vi "Actor Core.vi"(8 "error in":errorcluster, 11 "Nested in":refnum<class "MCLB_Template.lvclass">) -> (0 "error out":errorcluster, 3 "Actor out":refnum<class "Actor.lvclass">)   [LabVIEW 2021, in "MCLB_Template.lvclass"]
doc: "(<B>Filename</B>: Actor Framework.lvlib:Actor.lvclass:Actor Core.vi)\n\nReceives messages to the actor, reacts to them, and initiates any error handling that may shut the actor down.\n\nDescendant classes may override this VI to append parallel tasks for the actor to complete while it handles messages. Overrides use the Call Parent Method node."
uses:
  MCLB_Template.lvclass
  C:/Program Files (x86)/National Instruments/LabVIEW 2021/user.lib/John_Lib/AbstractActorTemplate/AbstractActorTemplate/UIActorTop.lvclass
  C:/Program Files (x86)/National Instruments/LabVIEW 2021/vi.lib/ActorFramework/Actor/Actor.lvclass
  <vilib>/ActorFramework/Actor/Actor.lvclass
  <userlib>/John_Lib/Control_Lib/MCLB_Lib/MCLB_Lib.lvclass
  <vilib>/Utility/miscctls.llb/LVRowAndColumnTypeDef.ctl
  MCLB_Template.lvclass/MCLB_Template.ctl
  <vilib>/ActorFramework/Actor/Actor.lvclass/Actor.ctl
  <vilib>/ActorFramework/Message Enqueuer/Message Enqueuer.lvclass/Message Enqueuer.ctl
  <vilib>/Utility/miscctls.llb/LVPoint32TypeDef.ctl
  <userlib>/John_Lib/Interfaces/MouseHandle Messages/Mouse Down Msg/Mouse Down Msg.lvclass/Mouse Down Msg.ctl
  <userlib>/John_Lib/Interfaces/MouseHandle Messages/Mouse RightDown Msg/Mouse RightDown Msg.lvclass/Mouse RightDown Msg.ctl
  <userlib>/John_Lib/Interfaces/Shortcut Menu Messages/Activation Msg/Activation Msg.lvclass/Activation Msg.ctl
  <userlib>/John_Lib/Interfaces/Shortcut Menu Messages/Menu Selection (User) Msg/Menu Selection (User) Msg.lvclass/Menu Selection (User) Msg.ctl
  <userlib>/John_Lib/Interfaces/MouseHandle Messages/Mouse Move Msg/Mouse Move Msg.lvclass/Mouse Move Msg.ctl
  <userlib>/John_Lib/Interfaces/MouseHandle Messages/Mouse UP Msg/Mouse UP Msg.lvclass/Mouse UP Msg.ctl
  <vilib>/ActorFramework/Message Enqueuer/Init from Existing Queue.vi
  <vilib>/ActorFramework/Message Enqueuer/Enqueue.vi
  <vilib>/ActorFramework/Stop Msg/Stop Msg.lvclass
  C:/Program Files (x86)/National Instruments/LabVIEW 2021/vi.lib/ActorFramework/Message/Message.lvclass
  <userlib>/John_Lib/Interfaces/MouseHandle Messages/Mouse Down Msg/Mouse Down Msg.lvclass
  <userlib>/John_Lib/Interfaces/MouseHandle Messages/Mouse RightDown Msg/Mouse RightDown Msg.lvclass
  <userlib>/John_Lib/Interfaces/Shortcut Menu Messages/Activation Msg/Activation Msg.lvclass
  <userlib>/John_Lib/Interfaces/Shortcut Menu Messages/Menu Selection (User) Msg/Menu Selection (User) Msg.lvclass
  <userlib>/John_Lib/Interfaces/MouseHandle Messages/Mouse Move Msg/Mouse Move Msg.lvclass
  <userlib>/John_Lib/Interfaces/MouseHandle Messages/Mouse UP Msg/Mouse UP Msg.lvclass
  <vilib>/ActorFramework/Message Priority Queue/Priority Enqueue.vi
  <vilib>/ActorFramework/Message Enqueuer/Message Enqueuer.lvclass
  <userlib>/John_Lib/AbstractActorTemplate/AbstractActorTemplate/UIActorTop.lvclass
panel:
  in  "MCLB":i32[](listbox)
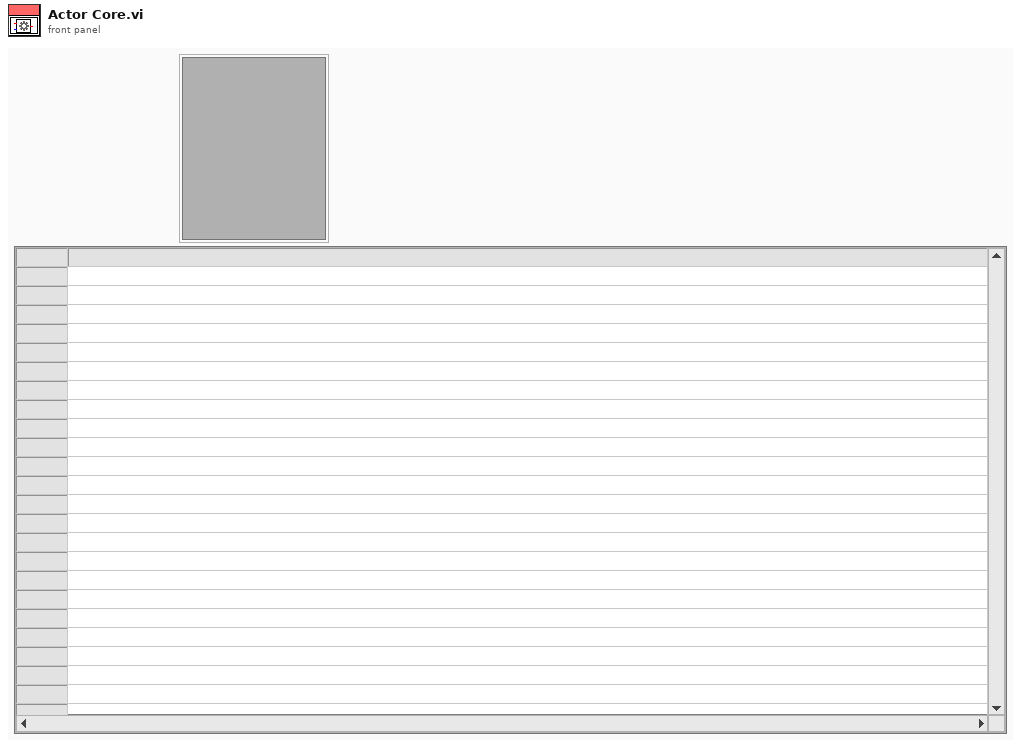
[diagram p1: front panel]
types:
  T1 = typedef "LVRowAndColumnTypeDef.ctl" = cluster{"Row":i32, "Column":i32}
  T2 = typedef "LVPoint32TypeDef.ctl" = cluster{"Horizontal":i32, "Vertical":i32}
  T3 = typedef "MouseButton.ctl" = enum16{"Idle", "Left", "Right", "Middle"}
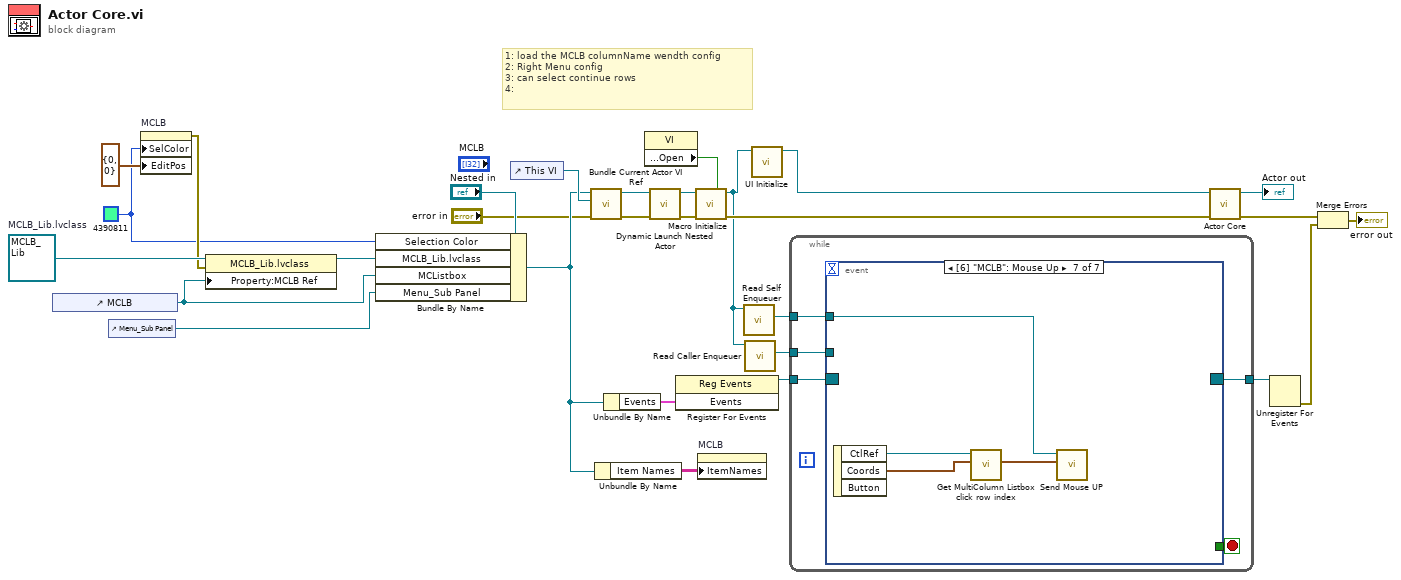
[diagram p0: block diagram]
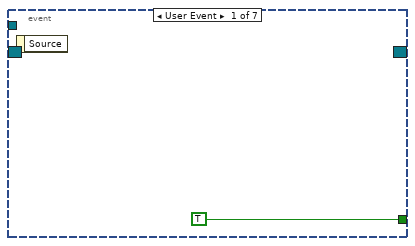
[diagram p2: hidden frame]
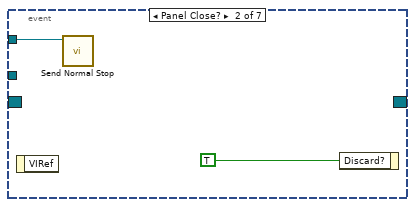
[diagram p3: hidden frame]
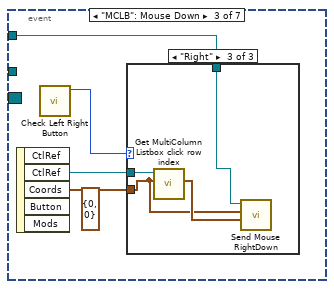
[diagram p4: hidden frame]
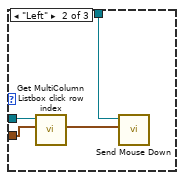
[diagram p6: hidden frame]
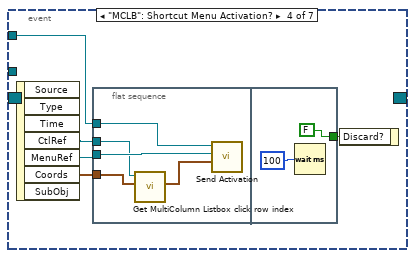
[diagram p7: hidden frame]
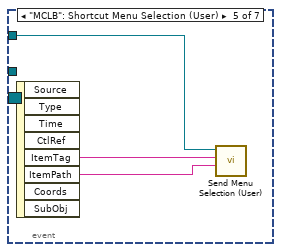
[diagram p8: hidden frame]
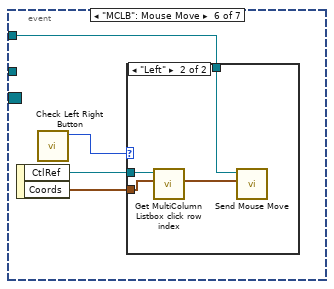
[diagram p9: hidden frame]
diagram:
  w12 = refnum<class "MCLB_Lib.lvclass"> refnum  # MCLB_Lib.lvclass
  w3 = u32 4390811 ("OK")
  # "1: load the MCLB columnName wendth config\n2: Right Menu config\n3: can select continue rows\n4:"
  n1 = control-ref of="MCLB"() -> (w10:refnum<vi>)
  n2 = control-ref of="Menu_Sub Panel"() -> (w9:refnum<vi>)
  n3 = property on="MCLB" class="MCListbox (strict)"("SelColor"=w3, "EditPos"=T1 {"Row"=0, "Column"=0} ("Edit Position")) -> (error out=w7:errorcluster)  [unwired: 2 in, 1 out]
  n4 = property class="MCLB_Lib.lvclass"(reference=w12, error in=w7, "Property:MCLB Ref"=w10) -> (reference out=w11:refnum<class "MCLB_Lib.lvclass">)  [unwired: 1 out]
  n5 = Bundle By Name(cluster="Nested in", "Selection Color"=w3, "MCLB_Lib.lvclass"=w11, "MCListbox"=w10, "Menu_Sub Panel"=w9) -> (w6:refnum<class "MCLB_Template.lvclass">)
  n6 = control-ref of="This VI"() -> (w13:refnum<vi>)
  n7 = call <userlib>:"Bundle Current Actor VI Ref.vi"("error in (no error)"="error in", "This VI"=w13, "UI ActorTop in"=w6) -> ("error out"=w14:errorcluster, "UI ActorTop out"=w15:refnum<class "MCLB_Template.lvclass">)  [unwired: 5 in, 2 out]
  n8 = Unbundle By Name(w6) -> ("Item Names"=w2:string[][])
  n9 = Unbundle By Name(w6) -> ("Events"=w27:cluster{"Stop":refnum<user-event>})
  n10 = property class="VI"() -> ("Front Panel.Open"=w22:bool)  [unwired: 2 in, 2 out]
  n11 = call-dynamic "Dynamic Launch Nested Actor.vi"("error in (no error)"=w14, "UI ActorTop in"=w15) -> ("error out"=w23:errorcluster, "UI ActorTop out"=w24:refnum<class "MCLB_Template.lvclass">)  [unwired: 8 in]
  n12 = register-events ("Main Register for Events")(w27) -> (reference out=w28:refnum<event-registration>)  [unwired: 2 in, 1 out]
  n13 = call-dynamic "Macro Initialize.vi"("Front Panel Window:Open"=w22, "error in (no error)"=w23, "UI ActorTop in"=w24) -> ("error out"=w18:errorcluster, "UI ActorTop out"=w5:refnum<class "MCLB_Template.lvclass">)  [unwired: 7 in]
  n14 = property on="MCLB" class="MCListbox (strict)"("ItemNames"=w2) -> ()  [unwired: 2 in, 2 out]
  n15 = call <vilib>:"Read Self Enqueuer.vi"("Actor"=w5) -> ("Self Enqueuer"=w25:refnum<class "Message Enqueuer.lvclass">)  [unwired: 10 in]
  n16 = call <vilib>:"Read Caller Enqueuer.vi"("Actor"=w5) -> ("Caller Enqueuer"=w17:refnum<class "Message Enqueuer.lvclass">)  [unwired: 10 in]
  n17 = call-dynamic "UI Initialize.vi"("UI ActorTop in"=w5) -> ("UI ActorTop out"=w4:refnum<class "MCLB_Template.lvclass">)  [unwired: 9 in, 1 out]
  n18 = while {
    tunnel: w28 -> [w34]
    tunnel: [w32] -> w26
    tunnel: w25 -> [w31]
    tunnel: w17 -> [w30]
    stop <- w33 stop-if-true
    n19 = event "UI Events" shown="[6] \"MCLB\": Mouse Up" {
      selector: w34 -> [_ _ _ _ _ _ _]
      dyn-events: [_ _ _ _ _ _ _] -> w32
      timeout: _ -> [_ _ _ _ _ _ _]
      tunnel: [TRUE _ _ _ _ _ _] -> w33
      tunnel: w31 -> [_ w36 w38 w54 w62 w65 w74]
      tunnel: w30 -> [_ _ _ _ _ _ _]
      event User Event {
        n20 = event-data() -> ()  [unwired: 1 in, 1 out]
      }
      event Panel Close? {
        n21 = event-data() -> ()  [unwired: 1 in, 1 out]
        n22 = call <vilib>:"Send Normal Stop.vi"("Message Enqueuer"=w36) -> ()  [unwired: 10 in, 1 out]
        n23 = event-data("Discard?"=TRUE) -> ()  [unwired: 1 in, 1 out]
      }
      event "MCLB": Mouse Down {
        (unwired) T2 {"Horizontal"=0, "Vertical"=0} ("Coords")
        n24 = event-data() -> ("CtlRef"=w41:refnum<vi>, "Coords"=w40:T2)  [unwired: 1 in, 3 out]
        n25 = call <userlib>:"Check Left Right Button.vi"() -> ("MouseButton"=w39:T3)  [unwired: 8 in, 3 out]
        n26 = case shown="\"Right\"" w39 {
          tunnel: w41 -> [_ w45 w49]
          tunnel: w40 -> [_ w44 w46]
          tunnel: w38 -> [_ w42 w48]
          frame "Idle", Default {
          }
          frame "Left" {
            n27 = call <userlib>:"Get MultiColumn Listbox click row index.vi"("Coords"=w44, "CtlRef"=w45) -> ("Cell Position"=w43:T1)  [unwired: 5 in, 4 out]
            n28 = call <userlib>:"Send Mouse Down.vi"("Cell Position"=w43, "Message Enqueuer"=w42) -> ()  [unwired: 8 in, 2 out]
          }
          frame "Right" {
            n29 = call <userlib>:"Get MultiColumn Listbox click row index.vi"("Coords"=w46, "CtlRef"=w49) -> ("Cell Position"=w47:T1)  [unwired: 5 in, 4 out]
            n30 = call <userlib>:"Send Mouse RightDown.vi"("Cell Position"=w47, "Coords"=w46, "Message Enqueuer"=w48) -> ()  [unwired: 7 in, 2 out]
          }
        }
      }
      event "MCLB": Shortcut Menu Activation? {
        n31 = event-data() -> ("CtlRef"=w50:refnum<vi>, "MenuRef"=w53:refnum<k9>, "Coords"=w51:T2)  [unwired: 1 in, 4 out]
        n32 = flat-sequence {
          tunnel: w54 -> [w59]
          tunnel: w53 -> [w56]
          tunnel: w51 -> [w57]
          tunnel: w50 -> [w55]
          tunnel: [FALSE ("Discard?")] -> w52
          frame #0 {
            n33 = call <userlib>:"Get MultiColumn Listbox click row index.vi"("Coords"=w57, "CtlRef"=w55) -> ("Cell Position"=w58:T1)  [unwired: 5 in, 4 out]
            n34 = call <userlib>:"Send Activation.vi"("Cell Position"=w58, "MenuRef"=w56, "Message Enqueuer"=w59) -> ()  [unwired: 7 in, 2 out]
          }
          frame #1 {
            n35 = Wait (ms)(milliseconds to wait=u32 100) -> ()  [unwired: 1 out]
          }
        }
        n36 = event-data("Discard?"=w52) -> ()  [unwired: 1 in, 1 out]
      }
      event "MCLB": Shortcut Menu Selection (User) {
        n37 = event-data() -> ("ItemTag"=w63:string, "ItemPath"=w64:string)  [unwired: 1 in, 6 out]
        n38 = call <userlib>:"Send Menu Selection (User).vi"("ItemPath"=w64, "ItemTag"=w63, "Message Enqueuer"=w62) -> ()  [unwired: 7 in, 2 out]
      }
      event "MCLB": Mouse Move {
        n39 = event-data() -> ("CtlRef"=w68:refnum<vi>, "Coords"=w67:T2)  [unwired: 1 in]
        n40 = call <userlib>:"Check Left Right Button.vi"() -> ("MouseButton"=w66:T3)  [unwired: 8 in, 3 out]
        n41 = case shown="\"Left\"" w66 {
          tunnel: w68 -> [_ w72]
          tunnel: w67 -> [_ w71]
          tunnel: w65 -> [_ w69]
          frame "Idle", Default {
          }
          frame "Left" {
            n42 = call <userlib>:"Get MultiColumn Listbox click row index.vi"("Coords"=w71, "CtlRef"=w72) -> ("Cell Position"=w70:T1)  [unwired: 5 in, 4 out]
            n43 = call <userlib>:"Send Mouse Move.vi"("Cell Position"=w70, "Message Enqueuer"=w69) -> ()  [unwired: 8 in, 2 out]
          }
        }
      }
      event "MCLB": Mouse Up {
        n44 = event-data() -> ("CtlRef"=w76:refnum<vi>, "Coords"=w75:T2)  [unwired: 1 in, 1 out]
        n45 = call <userlib>:"Get MultiColumn Listbox click row index.vi"("Coords"=w75, "CtlRef"=w76) -> ("Cell Position"=w73:T1)  [unwired: 5 in, 4 out]
        n46 = call <userlib>:"Send Mouse UP.vi"("Cell Position"=w73, "Message Enqueuer"=w74) -> ()  [unwired: 8 in, 2 out]
      }
    }
  }
  n47 = call-parent "Actor Core.vi"("error in"=w18, "Actor in"=w4) -> ("error out"=w20:errorcluster, "Actor out"=→"Actor out":refnum<class "Actor.lvclass">)  [unwired: 8 in]
  n48 = Unregister For Events(event registration refnum=w26) -> (error out=w21:errorcluster)  [unwired: 1 in]
  n49 = Merge Errors(w20, w21) -> (→"error out":errorcluster)
